vi "request response test.vi"() -> (0 "error out":errorcluster)   [LabVIEW 2024]
uses:
  src/NATS Client/NATS Client.lvclass/NATS Client.ctl
  <vilib>/NATS/NATS Core/VIs/NATS CLOSE.vi
  src/NATS Client/get async stop notifier.vi
  src/NATS Client/Get Connection DVR.vi
  src/NATS Client/get subscriptions queue.vi
  src/NATS Client/Get subscription map.vi
  src/NATS Client/Get error queue.vi
  <vilib>/addons/_JKI Toolkits/Caraya/classes/Assert/Assert True.vi
  <vilib>/addons/_JKI Toolkits/Caraya/classes/Assert/Assert False.vi
  <vilib>/addons/_JKI Toolkits/Caraya/classes/Assert/Assert Equal Value and Type_Variant.vi
  src/NATS Subscription/NATS Subscription.lvclass
  <vilib>/addons/_JKI Toolkits/Caraya/classes/Test/Test.lvclass
  src/NATS Client/NATS Client.lvclass
  <vilib>/addons/_JKI Toolkits/Caraya/classes/Assert/Assert.lvclass
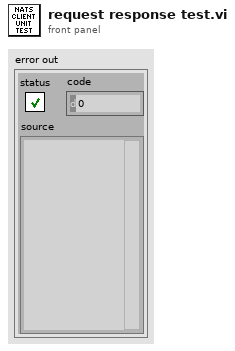
[diagram p1: front panel]
types:
  T1 = typedef "NATS Core.lvlib/nats message.ctl" = cluster{"subject":string, "payload":string, "sub id":string, "reply-to":string, "headers":string, "type":T2, "received":timestamp}
  T2 = typedef "NATS Core.lvlib/msg type.ctl" = enum16{"Undefined", "MSG", "HMSG", "+OK", "PING", "PONG", "-ERR", "INFO"}
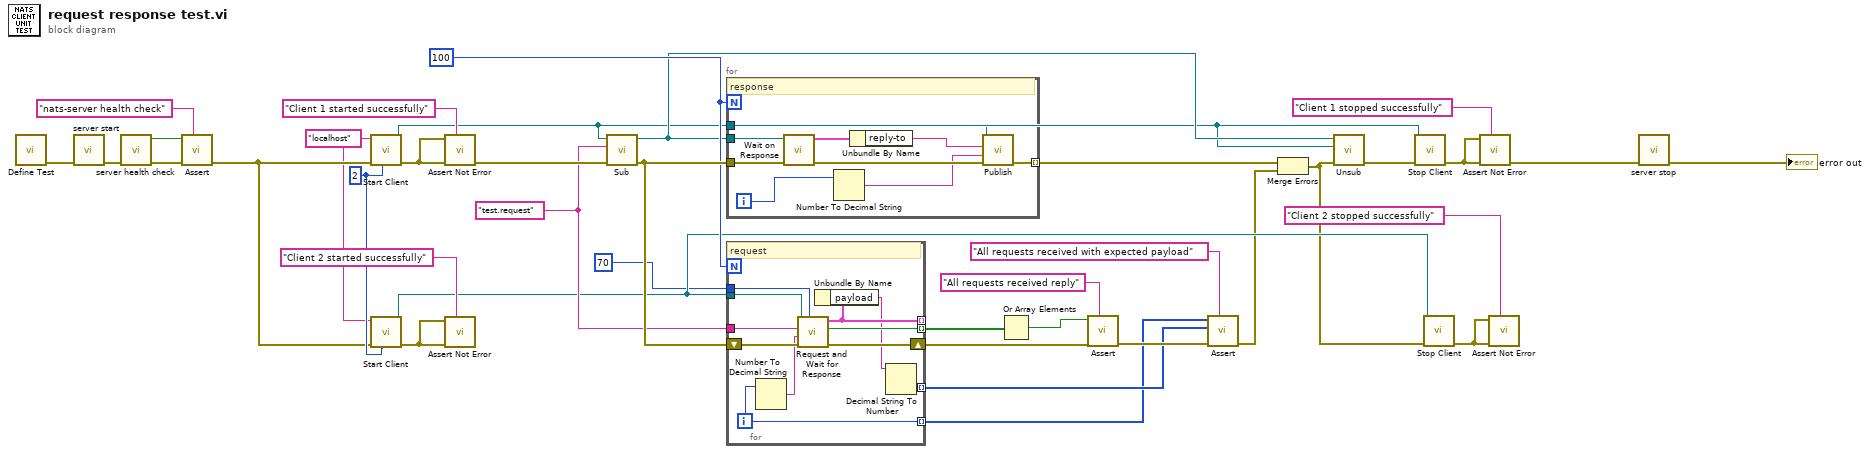
[diagram p0: block diagram]
diagram:
  w10 = 2 ("timeout ms (5)")
  w26 = 100
  w27 = "test.request"
  w2 = "localhost" ("address")
  n1 = call <vilib>:"Define Test.vi"() -> ("error out"=w9:errorcluster)  [unwired: 10 in, 1 out]
  n2 = call "server start.vi"("error in"=w9) -> ("error out"=w8:errorcluster)  [unwired: 10 in]
  n3 = call "server health check.vi"("error in"=w8) -> ("error out"=w7:errorcluster, "healthy"=w6:bool)  [unwired: 9 in]
  n4 = call-poly <vilib>:"Assert.vi"("Label"="nats-server health check", "error in (no error)"=w7, "True?"=w6) -> ("error out"=w4:errorcluster)  [unwired: 7 in, 1 out]
  n5 = call "Start Client.vi"("timeout ms (5)"=w10, "error in"=w4, "address"=w2) -> ("error out"=w38:errorcluster, "NATS Client out"=w22:refnum<class "NATS Client.lvclass">)  [unwired: 7 in]
  n6 = call "Start Client.vi"("timeout ms (5)"=w10, "error in"=w4, "address"=w2) -> ("error out"=w35:errorcluster, "NATS Client out"=w23:refnum<class "NATS Client.lvclass">)  [unwired: 7 in]
  n7 = call <vilib>:"Assert Not Error.vi"("Label"="Client 1 started successfully", "error in (no error)"=w38, "Not Error?"=w38) -> ("error out"=w34:errorcluster)  [unwired: 7 in, 1 out]
  n8 = call <vilib>:"Assert Not Error.vi"("Label"="Client 2 started successfully", "error in (no error)"=w35, "Not Error?"=w35) -> ()  [unwired: 7 in, 2 out]
  n9 = call "Sub.vi"("error in"=w34, "subject"=w27, "NATS Client"=w22) -> ("error out"=w31:errorcluster, "NATS Subscription"=w25:refnum<class "NATS Subscription.lvclass">)  [unwired: 7 in]
  n10 = for {
    N: w26 -> [_]
    tunnel: w25 -> [w46]
    tunnel: w22 -> [w44]
    tunnel: w31 -> [w47]
    tunnel: [w39] -> w19 mode=indexing
    i -> [w41]
    # "response"
    n11 = call "Wait on Response.vi"("error in"=w47, "NATS Subscriber in"=w46) -> ("error out"=w45:errorcluster, "nats message"=w43:T1)  [unwired: 7 in, 1 out]
    n12 = Number To Decimal String(number=w41) -> (decimal integer string=w40:string)  [unwired: 1 in]
    n13 = Unbundle By Name(w43) -> ("reply-to"=w42:string)
    n14 = call "Publish.vi"("error in"=w45, "payload"=w40, "subject"=w42, "NATS Client.lvlib:NATS Client.lvclass"=w44) -> ("error out"=w39:errorcluster)  [unwired: 7 in]
  }
  n15 = for {
    N: w26 -> [_]
    tunnel: w23 -> [w56]
    tunnel: w27 -> [w55]
    shift-right: [w57] -> w17
    shift-left: w31 -> [w58]
    tunnel: [w54] -> w21 mode=indexing
    tunnel: [w53] -> _ mode=indexing
    tunnel: [w50] -> w15 mode=indexing
    tunnel: [w49] -> w14 mode=indexing
    tunnel: 70 ("timeout in ms (-1)") -> [w48]
    i -> [w49]
    # "request"
    n16 = Number To Decimal String(number=w49) -> (decimal integer string=w52:string)  [unwired: 1 in]
    n17 = call "Request and Wait for Response.vi"("timeout in ms (-1)"=w48, "error in"=w58, "payload"=w52, "subject"=w55, "NATS Client in"=w56) -> ("error out"=w57:errorcluster, "time out"=w54:bool, "nats message"=w53:T1)  [unwired: 4 in]
    n18 = Unbundle By Name(w53) -> ("payload"=w51:string)
    n19 = Decimal String To Number(string=w51) -> (number=w50:i32)  [unwired: 2 in, 1 out]
  }
  n20 = Or Array Elements(Boolean array=w21) -> (logical OR=w20:bool)
  n21 = call-poly <vilib>:"Assert.vi"("Label"="All requests received reply", "error in (no error)"=w17, "False?"=w20) -> ("error out"=w18:errorcluster)  [unwired: 7 in, 1 out]
  n22 = call-poly <vilib>:"Assert.vi"("Label"="All requests received with expected payload", "error in (no error)"=w18, "Actual"=w15, "Expected"=w14) -> ("error out"=w12:errorcluster)  [unwired: 6 in, 1 out]
  n23 = Merge Errors(w19, w12) -> (w11:errorcluster)
  n24 = call "Unsub.vi"("error in"=w11, "NATS Client"=w22, "NATS Subscription"=w25) -> ("error out"=w33:errorcluster)  [unwired: 7 in, 1 out]
  n25 = call "Stop Client.vi"("error in"=w33, "NATS Client"=w22) -> ("error out"=w37:errorcluster)  [unwired: 9 in]
  n26 = call "Stop Client.vi"("error in"=w11, "NATS Client"=w23) -> ("error out"=w32:errorcluster)  [unwired: 9 in]
  n27 = call <vilib>:"Assert Not Error.vi"("Label"="Client 1 stopped successfully", "error in (no error)"=w37, "Not Error?"=w37) -> ("error out"=w36:errorcluster)  [unwired: 7 in, 1 out]
  n28 = call <vilib>:"Assert Not Error.vi"("Label"="Client 2 stopped successfully", "error in (no error)"=w32, "Not Error?"=w32) -> ()  [unwired: 7 in, 2 out]
  n29 = call "server stop.vi"("error in"=w36) -> ("error out"=→"error out":errorcluster)  [unwired: 10 in]
